vi "Register Game Start Event.vi"(8 "error in (no error)":errorcluster, 10 "Game Start":refnum<user-event>, 11 "Game Config Panel in":refnum<class "Game Config Panel.lvclass">) -> (0 "error out":errorcluster, 3 "Game Config Panel out":refnum<class "Game Config Panel.lvclass">)   [LabVIEW 2020, in "SB App.lvlib" / "Game Config Panel.lvclass"]
uses:
  Game Config Panel.lvclass
  Game Start Data.ctl
  Game Config Panel.lvclass/Game Config Panel.ctl
  SB App.lvlib
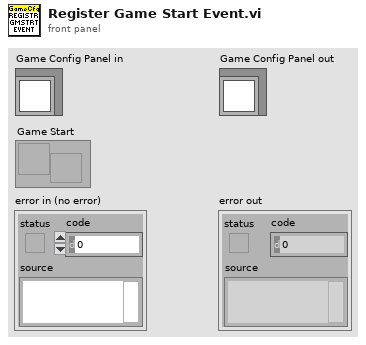
[diagram p1: front panel]
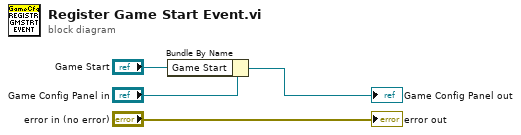
[diagram p0: block diagram]
diagram:
  n1 = Bundle By Name(cluster="Game Config Panel in", "Game Start"="Game Start") -> (→"Game Config Panel out":refnum<class "Game Config Panel.lvclass">)
  "error out" <- "error in (no error)"
